vi "Query Status Register.vi"(8 "error in (no error)":errorcluster, 11 "Acopian in":refnum<class "Acopian.lvclass">) -> (0 "error out":errorcluster, 3 "Acopian out":refnum<class "Acopian.lvclass">)   [LabVIEW 2019, in "Acopian.lvlib" / "Acopian.lvclass"]
doc: "Child classes must override this VI:\n\nThis VI is the device specific query of the supply's status registers. \nThe return values are: \n\nThe implementation must read status registers and push the status register values to private data for:\nOCP Flag, OVP Flag, Interlock Flag, Output Flag into the private data arrays of the power supply class."
uses:
  Library/Acopian.lvclass
  builds/Instruments/PowerSupply.lvlibp/Library/PowerSupply.lvclass
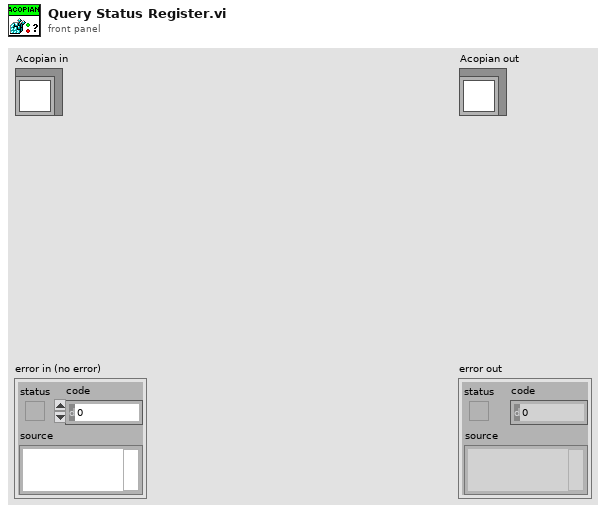
[diagram p1: front panel]
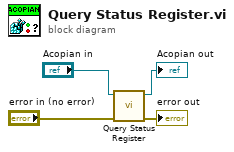
[diagram p0: block diagram]
diagram:
  n1 = call-parent "Query Status Register.vi"("error in (no error)"="error in (no error)", "PowerSupply in"="Acopian in") -> ("error out"=→"error out":errorcluster, "PowerSupply out"=→"Acopian out":refnum<class "Acopian.lvclass">)  [unwired: 8 in]
